vi "Test Power Shell.vi"   [LabVIEW 2018]
uses:
  Microsoft.PowerShell.Commands.Utility
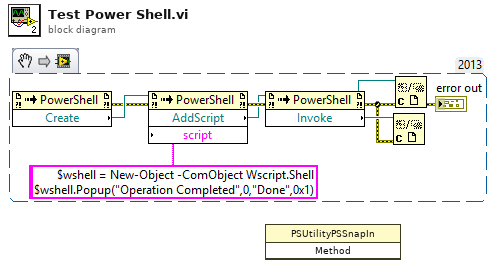
[diagram p0: block diagram]
diagram:
  n1 = invoke class="PSUtilityPSSnapIn" method=#-1() -> ()  [unwired: 3 in, 3 out]
